vi "SIMDMM_Timestamp Add.vi"(1 "y":timestamp format="%<%X\n%x>T", 2 "x":timestamp format="%<%X\n%x>T") -> (0 "x + y":timestamp format="%<%X\n%x>T")   [LabVIEW 2019]
uses:
  SIMDMM_I128 Timestamp.ctl
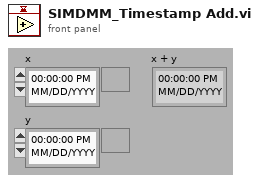
[diagram p1: front panel]
types:
  T1 = typedef "SIMDMM_I128 Timestamp.ctl" = cluster{"high":i32, "mid high":u32, "mid low":u32, "low":u32}
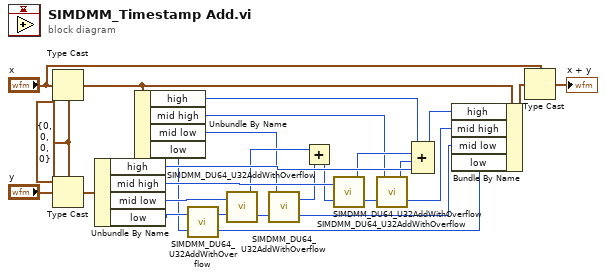
[diagram p0: block diagram]
diagram:
  w2 = T1 {"high"=0, "mid high"=0, "mid low"=0, "low"=0} ("timestamp")
  n1 = Type Cast(type=w2, x="x") -> (*(type *) &x=w3:T1)
  n2 = Type Cast(type=w2, x="y") -> (*(type *) &x=w4:T1)
  n3 = Unbundle By Name(w4) -> ("high"=w24:i32, "mid high"=w25:u32, "mid low"=w26:u32, "low"=w27:u32)
  n4 = Unbundle By Name(w3) -> ("high"=w16:i32, "mid high"=w15:u32, "mid low"=w10:u32, "low"=w7:u32)
  n5 = call "SIMDMM_DU64_U32AddWithOverflow.vi"("input 2"=w7, "input 1"=w27) -> ("output"=w19:u32, "overflow"=w8:u32)
  n6 = call "SIMDMM_DU64_U32AddWithOverflow.vi"("input 2"=w8, "input 1"=w26) -> ("output"=w9:u32, "overflow"=w12:u32)
  n7 = call "SIMDMM_DU64_U32AddWithOverflow.vi"("input 2"=w9, "input 1"=w10) -> ("output"=w20:u32, "overflow"=w11:u32)
  n8 = Add(x=w12, y=w11) -> (x+y=w13:u32)
  n9 = call "SIMDMM_DU64_U32AddWithOverflow.vi"("input 2"=w13, "input 1"=w25) -> ("output"=w14:u32, "overflow"=w18:u32)
  n10 = call "SIMDMM_DU64_U32AddWithOverflow.vi"("input 2"=w14, "input 1"=w15) -> ("output"=w21:u32, "overflow"=w17:u32)
  n11 = Compound Arithmetic op=ADD(w16, w18, w17, w24) -> (w22:u32)
  n12 = Bundle By Name(cluster=w3, "high"=w22, "mid high"=w21, "mid low"=w20, "low"=w19) -> (w23:T1)
  n13 = Type Cast(type="x", x=w23) -> (*(type *) &x=→"x + y":timestamp)
